vi "display.vi"(8 "error in (no error)":errorcluster, 11 "DisplayElement.lvclass":refnum<class "DisplayElement.lvclass">) -> (0 "error out":errorcluster, 3 "DisplayElement.lvclass 2":refnum<class "DisplayElement.lvclass">)   [LabVIEW 2020, in "DisplayElement.lvclass"]
uses:
  DisplayElement.lvclass
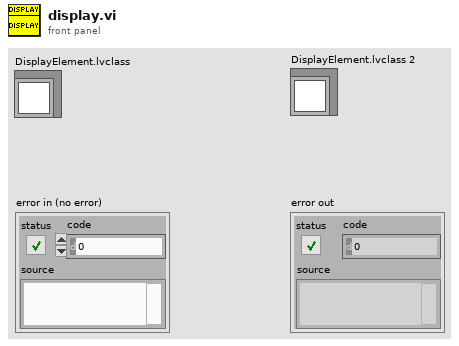
[diagram p1: front panel]
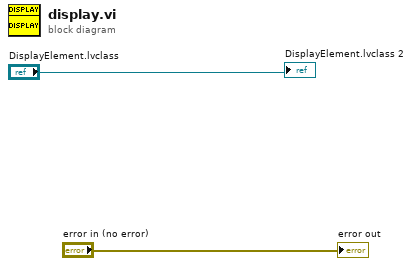
[diagram p0: block diagram]
diagram:
  "DisplayElement.lvclass 2" <- "DisplayElement.lvclass"
  "error out" <- "error in (no error)"
